vi "Get_bounding_box_for_object_at_coords.vi"(7 "Treat size as Radius (F)?":bool, 8 "Error In":errorcluster, 9 "Integer output (F)?":bool, 10 "Object Size, pix":cluster{"W":dbl, "H":dbl}, 11 "Object Coords, pix":cluster{"X":dbl, "Y":dbl}) -> (0 "Error Out":errorcluster, 3 "Object Bounding Box":T1)   [LabVIEW 2018, in "Cage Diagram.lvlib"]
uses:
  Cage Diagram.lvlib
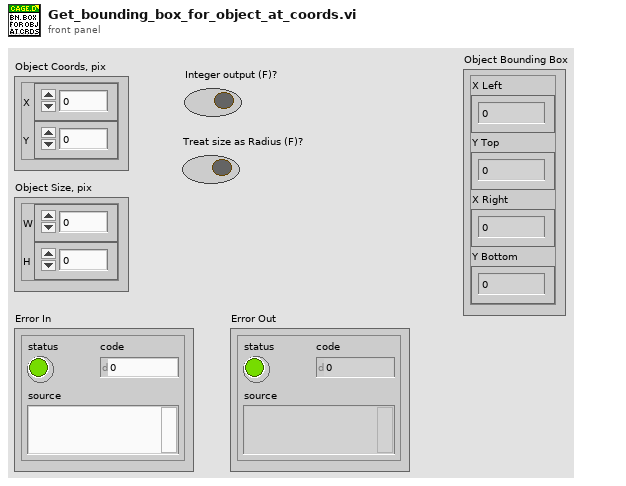
[diagram p1: front panel]
types:
  T1 = cluster{"X Left":dbl, "Y Top":dbl, "X Right":dbl, "Y Bottom":dbl}
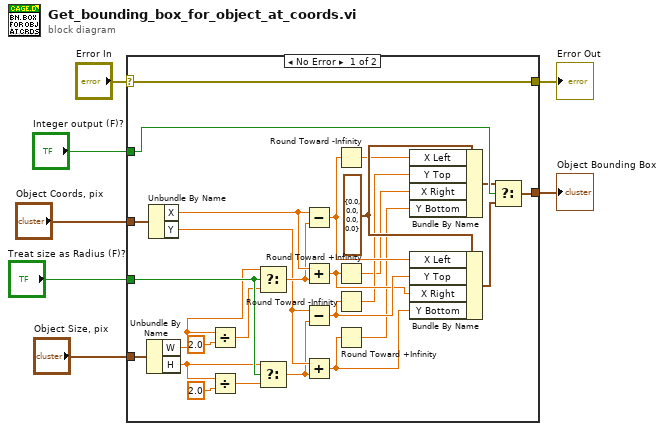
[diagram p0: block diagram]
diagram:
  n1 = case shown="No Error" "Error In" {
    selector: "Error In" -> [w25 w35]
    tunnel: [w25 w35] -> w6
    tunnel: "Treat size as Radius (F)?" -> [w28 _]
    tunnel: "Integer output (F)?" -> [w19 _]
    tunnel: "Object Coords, pix" -> [w34 _]
    tunnel: "Object Size, pix" -> [w33 _]
    tunnel: [w20 _] -> w1
    frame No Error {
      w17 = T1 {"X Left"=0.0, "Y Top"=0.0, "X Right"=0.0, "Y Bottom"=0.0} ("Object Bounding Box")
      n2 = Unbundle By Name(w33) -> ("W"=w23:dbl, "H"=w22:dbl)
      n3 = Unbundle By Name(w34) -> ("X"=w32:dbl, "Y"=w27:dbl)
      n4 = Divide(x=w23, y=2.0 ("x")) -> (x/y=w24:dbl)
      n5 = Divide(x=w22, y=2.0 ("x")) -> (x/y=w21:dbl)
      n6 = Select(t=w23, s=w28, f=w24) -> (s? t:f=w31:dbl)
      n7 = Select(t=w22, s=w28, f=w21) -> (s? t:f=w26:dbl)
      n8 = Subtract(x=w32, y=w31) -> (x-y=w15:dbl)
      n9 = Add(x=w32, y=w31) -> (x+y=w13:dbl)
      n10 = Subtract(x=w27, y=w26) -> (x-y=w14:dbl)
      n11 = Add(x=w27, y=w26) -> (x+y=w12:dbl)
      n12 = Round Toward -Infinity(1:w15) -> (0:w11:dbl)
      n13 = Round Toward +Infinity(x=w13) -> (ceil(x): smallest int >= x=w9:dbl)
      n14 = Round Toward -Infinity(1:w14) -> (0:w10:dbl)
      n15 = Round Toward +Infinity(x=w12) -> (ceil(x): smallest int >= x=w8:dbl)
      n16 = Bundle By Name(cluster=w17, "X Left"=w11, "Y Top"=w10, "X Right"=w9, "Y Bottom"=w8) -> (w16:T1)
      n17 = Bundle By Name(cluster=w17, "X Left"=w15, "Y Top"=w14, "X Right"=w13, "Y Bottom"=w12) -> (w18:T1)
      n18 = Select(t=w16, s=w19, f=w18) -> (s? t:f=w20:T1)
    }
    frame Error {
    }
  }
  "Error Out" <- w6
  "Object Bounding Box" <- w1
